vi "Reserve Dependency.vi"(7 "Reserving Entity":refnum<class "SMO.lvclass">, 8 "error in (no error)":errorcluster, 9 "Lock Key (if no reserving entity)":string caption="LockKey", 11 "SMO":refnum<class "SMO.lvclass">) -> (0 "error out":errorcluster, 1 "reserved":bool, 3 "SMO out":refnum<class "SMO.lvclass">)   [LabVIEW 2013, in "SMO.lvclass"]
doc: "SMO terminal to be connected with the resource that is to be reserved.\nReserving Entity is to be the reference to the object that reserves the SMO."
uses:
  SMO.lvclass
  SMO.lvclass/SMO.ctl
  Typedefs/Reserve State--Enum.ctl
  Support/Attribute.Owner/Attribute.Owner.lvclass
panel:
  # "For instructions on how to use the JKI State Machine Objects, examples and video tutorials, visit:\nhttp://jki.net/state-machine-objects/\n\nJKI State Machine Objects™\nhttp://jki.net/state-machine-objects/\nCopyright (C) 2005-2015, JKI <info@jki.net>\nALL RIGHTS RESERVED"
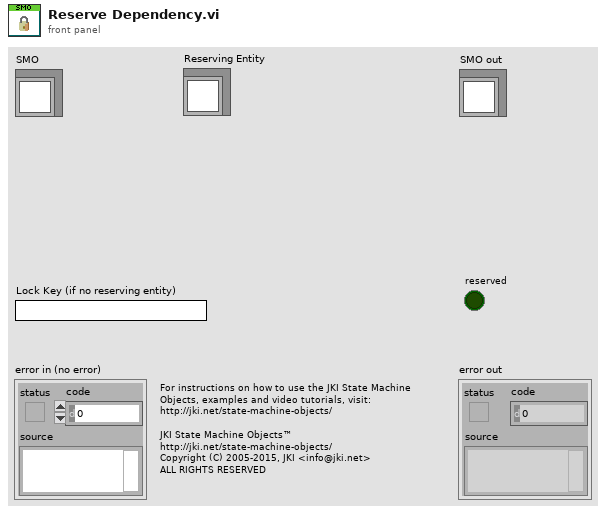
[diagram p1: front panel]
types:
  T1 = typedef "SMO.lvclass/Reserve State--Enum.ctl" = enum16{"Unreserved", "Reserved", "Self-locked"}
  T2 = typedef "SMO.lvclass/PrivateData--Ref.ctl" = refnum<data-value>
  T3 = typedef "SMO.lvclass/PrivateData--Cluster.ctl" = cluster{"Parent Call":T4, "Registered Processes":T5[], "Sync Notifier":refnum<notifier>, "Process Error Notifier":refnum<notifier>, "Protected Events":T6, "Public Events":T7, "SMO State":T8, "[Dependencies]":T9[], "[Attributes]":refnum<class "Attribute.lvclass">[], "Launcher Close":refnum<notifier>, "Caller Watchdog":refnum<queue>, "Accessibility":T10}
  T4 = typedef "SMO.lvclass/Parent Call--Enum.ctl" = enum16{"Allows parent to run", "Does not request parent to run"}
  T5 = typedef "SMO.lvclass/RegisteredProcessData--Cluster.ctl" = cluster{"Name":string, "Static VI Ref":refnum<vi>, "Running":bool, "NotifierRef":u32}
  T6 = typedef "SMO.lvclass/Protected Events.ctl" = cluster{"StopProcesses":refnum<user-event>, "AbortProcesses":refnum<user-event>, "Config Changed":refnum<user-event>, "Dependency":refnum<user-event>}
  T7 = typedef "SMO.lvclass/Public Events.ctl" = cluster{"Error":refnum<user-event>, "State":refnum<user-event>, "Reserve State":refnum<user-event>}
  T8 = typedef "SMO.lvclass/SMOState --Enum.ctl" = enum16{"unknown", "Created", "Started", "Stopped"}
  T9 = typedef "SMO.lvclass/SMO Dependency--Cluster.ctl" = cluster{"Dependency":refnum<class "SMO.lvclass">, "Level":string}
  T10 = typedef "SMO.lvclass/Accessibility--Cluster.ctl" = cluster{"Lock Key":string, "Reserve State":T1}
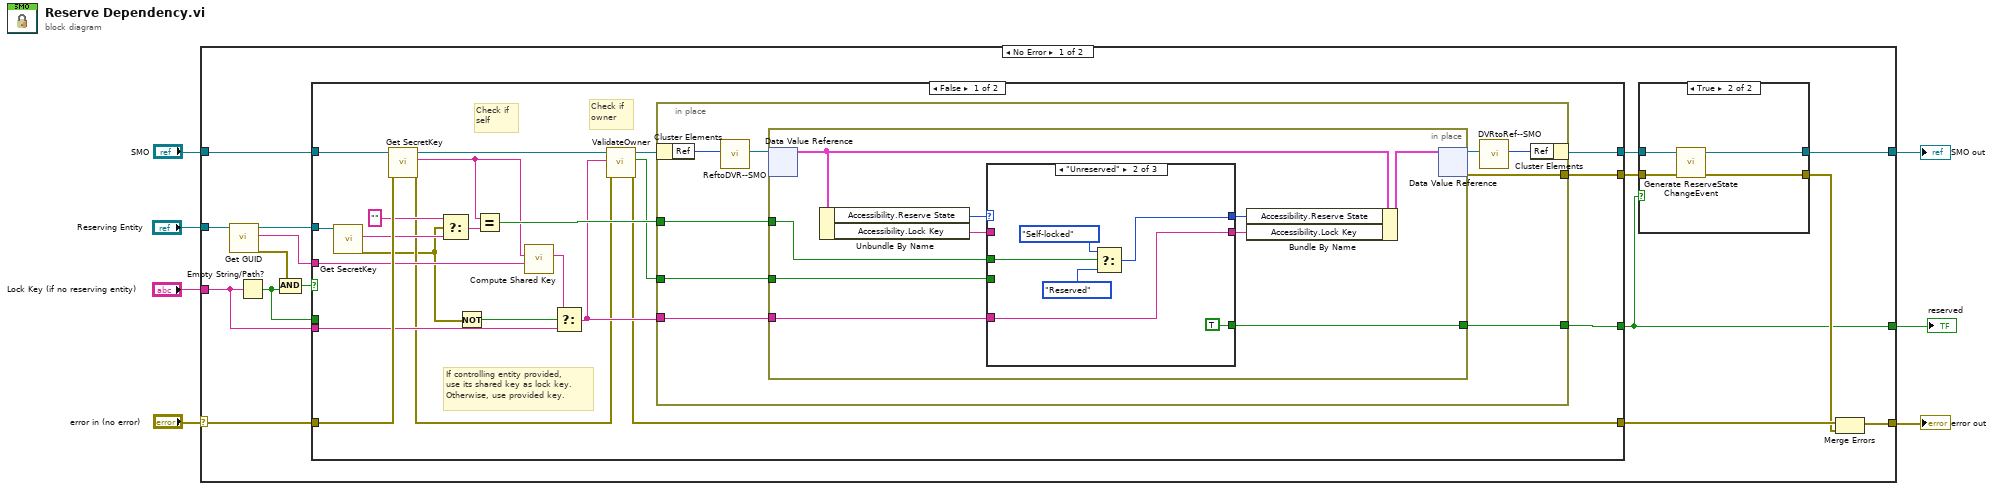
[diagram p0: block diagram]
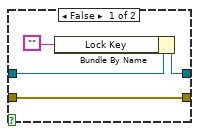
[diagram p2: hidden frame]
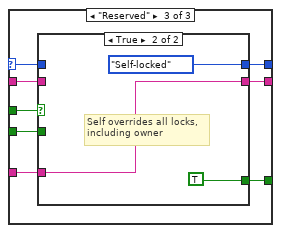
[diagram p4: hidden frame]
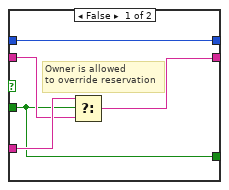
[diagram p5: hidden frame]
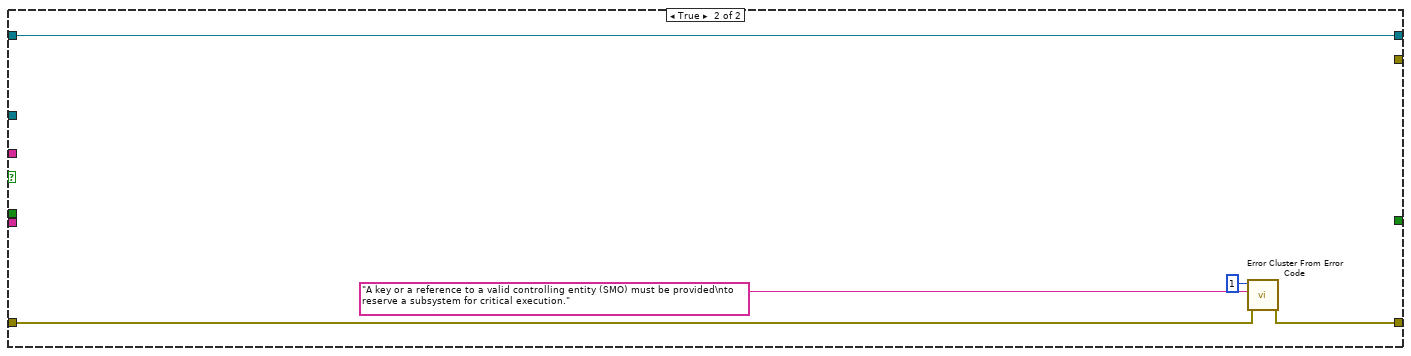
[diagram p6: hidden frame]
diagram:
  n1 = case shown="No Error" "error in (no error)" {
    selector: "error in (no error)" -> [w18 w103]
    tunnel: "SMO" -> [w17 w102]
    tunnel: [w11 w102] -> w6
    tunnel: [w23 w103] -> w5
    tunnel: "Reserving Entity" -> [w22 _]
    tunnel: "Lock Key (if no reserving entity)" -> [w15 _]
    tunnel: [w8 _] -> w1
    frame No Error {
      n2 = call "Get GUID.vi"("SMO"=w22) -> ("error out"=w21:errorcluster, "GUID"=w16:string, "SMO out"=w13:refnum<class "SMO.lvclass">)  [unwired: 8 in]
      n3 = Empty String/Path?(string/path=w15) -> (empty?=w14:bool)
      n4 = Compound Arithmetic op=AND(w21, w14) -> (w20:bool)
      n5 = case shown="False" w20 {
        tunnel: [w53 w101] -> w12
        tunnel: [w52 _] -> w9
        tunnel: w17 -> [w41 w101]
        tunnel: [w36 w99] -> w19
        tunnel: w18 -> [w51 w100]
        tunnel: w16 -> [w50 _]
        tunnel: w15 -> [w48 _]
        tunnel: w14 -> [_ _]
        tunnel: w13 -> [w47 _]
        tunnel: [w32 _] -> w8
        frame False {
          # "If controlling entity provided,\nuse its shared key as lock key.\nOtherwise, use provided key."
          # "Check if\nself"
          # "Check if\nowner"
          n6 = call "Get SecretKey.vi"("SMO"=w47) -> ("error out"=w34:errorcluster, "SecretKey"=w46:string)  [unwired: 8 in, 1 out]
          n7 = call "Get SecretKey.vi"("error in (no error)"=w51, "SMO"=w41) -> ("error out"=w37:errorcluster, "SecretKey"=w42:string, "SMO out"=w40:refnum<class "SMO.lvclass">)  [unwired: 7 in]
          n8 = Select(t="", s=w34, f=w46) -> (s? t:f=w44:string)
          n9 = Not(x=w34) -> (.not. x?=w33:bool)
          n10 = Equal?(x=w42, y=w44) -> (x = y?=w43:bool)
          n11 = call "Compute Shared Key.vi"("GUID"=w50, "SecretKey"=w42) -> ("Shared Key"=w49:string)  [unwired: 9 in]
          n12 = Select(t=w49, s=w33, f=w48) -> (s? t:f=w38:string)
          n13 = call "ValidateOwner.vi"("error in (no error)"=w37, "Shared Key"=w38, "SMO in"=w40) -> ("error out"=w36:errorcluster, "key matched"=w35:bool, "SMO out"=w39:refnum<class "SMO.lvclass">)  [unwired: 6 in]
          n14 = in-place {
            in-place-border: [w62] -> w52
            in-place-border: w38 -> [w57]
            in-place-border: w43 -> [w56]
            in-place-border: w35 -> [w55]
            in-place-border: [w54] -> w32
            n15 = in-place-cluster #1(w39) -> ("Ref"=w61:u32)
            n16 = call "ReftoDVR--SMO.vi"("Ref"=w61) -> ("Ref"=w60:T2)  [unwired: 10 in]
            n17 = in-place {
              in-place-border: w57 -> [w69]
              in-place-border: w56 -> [w66]
              in-place-border: w55 -> [w64]
              in-place-border: [w63] -> w54
              n18 = in-place-dvr #2(w60) -> (w71:T3)  [unwired: 1 out]
              n19 = Unbundle By Name(w71) -> ("Accessibility.Reserve State"=w72:T1, "Accessibility.Lock Key"=w65:string)
              n20 = case shown="\"Unreserved\"" w72 {
                selector: w72 -> [w74 _ w84]
                tunnel: w69 -> [_ w80 w85]
                tunnel: [w73 w80 w86] -> w68
                tunnel: [w74 w77 w87] -> w67
                tunnel: w66 -> [_ w76 w88]
                tunnel: w65 -> [w73 _ w83]
                tunnel: w64 -> [_ _ w82]
                tunnel: [_ TRUE ("key matched") w81] -> w63
                frame "Self-locked" {
                  # "Self-lock cannot be overwritten"
                }
                frame "Unreserved" {
                  n21 = Select(t=Reserve_State--Enum."Self-locked" ("Reserve State"), s=w76, f=Reserve_State--Enum."Reserved" ("Reserve State")) -> (s? t:f=w77:T1)
                }
                frame "Reserved" {
                  n22 = case shown="True" w88 {
                    tunnel: [w93 Reserve_State--Enum."Self-locked" ("Accessibility.Reserve State")] -> w87
                    tunnel: [w90 w95] -> w86
                    tunnel: w85 -> [w92 w95]
                    tunnel: w84 -> [w93 _]
                    tunnel: w83 -> [w91 _]
                    tunnel: w82 -> [w89 _]
                    tunnel: [w89 TRUE] -> w81
                    frame False {
                      # "Owner is allowed\nto override reservation"
                      n23 = Select(t=w92, s=w89, f=w91) -> (s? t:f=w90:string)
                    }
                    frame True {
                      # "Self overrides all locks, \nincluding owner"
                    }
                  }
                }
              }
              n24 = Bundle By Name(cluster=w71, "Accessibility.Reserve State"=w67, "Accessibility.Lock Key"=w68) -> (w70:T3)
              n25 = in-place-dvr #2(w70) -> (w59:T2, w62:errorcluster)
            }
            n26 = call "DVRtoRef--SMO.vi"("Ref"=w59) -> ("Ref"=w58:u32)  [unwired: 10 in]
            n27 = in-place-cluster #1("Ref"=w58) -> (w53:refnum<class "SMO.lvclass">)
          }
        }
        frame True {
          n28 = call <vilib>:"Error Cluster From Error Code.vi"("error in (no error)"=w100, "error message (\"\")"="A key or a reference to a valid controlling entity (SMO) must be provided\nto reserve a subsystem for critical execution." ("error message (\"\")"), "error code (0)"=1) -> ("error out"=w99:errorcluster)  [unwired: 6 in]
        }
      }
      n29 = case shown="True" w8 {
        tunnel: w12 -> [w26 w31]
        tunnel: [w25 w29] -> w11
        tunnel: [w27 w28] -> w10
        tunnel: w9 -> [w27 w30]
        frame False {
          n30 = Bundle By Name(cluster=w26, "Lock Key"="") -> (w25:refnum<class "SMO.lvclass">)
        }
        frame True {
          n31 = call "Generate ReserveState ChangeEvent.vi"("error in (no error)"=w30, "SMO in"=w31) -> ("error out"=w28:errorcluster, "SMO out"=w29:refnum<class "SMO.lvclass">)  [unwired: 8 in]
        }
      }
      n32 = Merge Errors(w19, w10) -> (w23:errorcluster)
    }
    frame Error {
    }
  }
  "error out" <- w5
  "SMO out" <- w6
  "reserved" <- w1
